vi "CleanHandler.constructor.vi"(0 "name":string, 2 "data in":string, 5 "error in(no error)":errorcluster) -> (14 "i ref out":refnum<vi>, 16 "data out":string, 19 "error out":errorcluster)   [LabVIEW 2014, in "CleanHandler.lvlib"]
doc: "A class handling a couple of DS345 (or a similar AFG) objects for sideband free cleaning by dipole excitation in the precision trap. Most of the DS345 are used to output a sine wave at the desired frequency. The amplitude of these DS345 is modulated by a Gaussian waveform that is generated by the first DS345 in the list of used devices. An instance of the CleanHandler instantiates its function generators when it is created. The function generators to be used are specified in the database.\n\nauthor: Dietrich Beck, GSI\n\nLicense Agreement for this software:\n\nCopyright (C)\nGesellschaft für Schwerionenforschung, GSI\nPlanckstr. 1\n64291 Darmstadt\nGermany\n\nContact: D.Beck@gsi.de \n\nThis program is free software; you can redistribute it and/or modify it under the terms of the \nGNU General Public License as published by the Free Software Foundation; either version 2 of \nthe license, or (at your option) any later version.\n\nThis program is distributed in the hope that it will be useful, but WITHOUT ANY WARRANTY; \nwithout even the implied warranty of MERCHANTABILITY or FITNESS FOR A PARTICULAR PURPOSE. See the GNU General License for more details (http://www.gnu.org).\n\nGesellschaft für Schwerionenforschung, GSI\nPlanckstr. 1, 64291 Darmstadt, Germany\nFor all questions and ideas contact: M.Richter@gsi.de, H.Brand@gsi.de or D.Beck@gsi.de.\nLast update: 16-JUN-2004"
uses:
  CleanHandler.lvlib
  CS_Core/BaseProcess/BaseProcess.lvlib
  CS_Core/CSSystem/CSSystemLib/CSSystemLib.lvlib
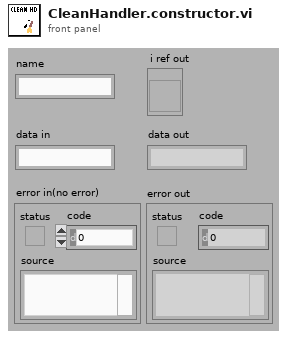
[diagram p1: front panel]
types:
  T1 = enum16{"SetAttribute", "GetAttribute", "CreateAttribute", "DestroyAttribute", "DestroyAllAtributes"}
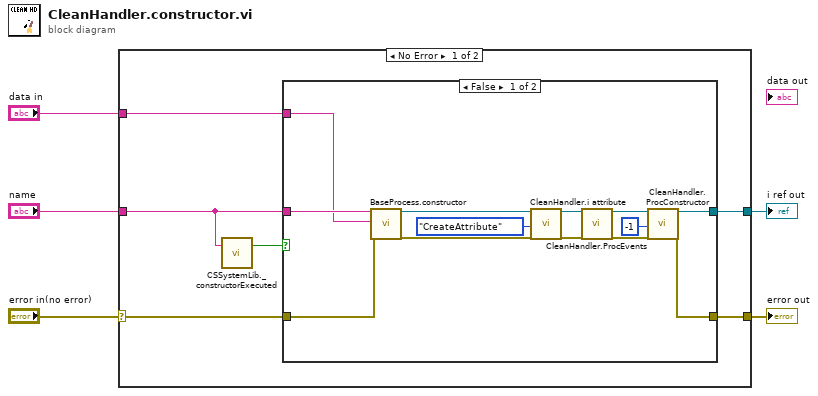
[diagram p0: block diagram]
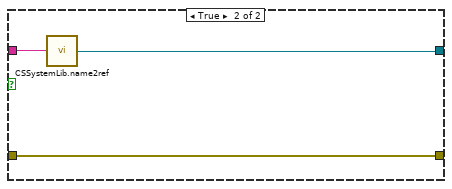
[diagram p2: hidden frame]
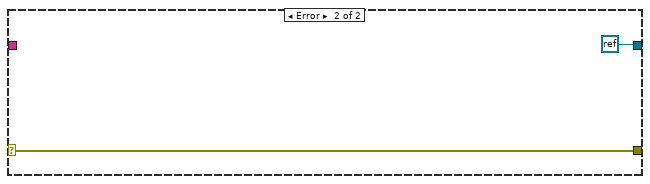
[diagram p3: hidden frame]
diagram:
  n1 = case shown="No Error" "error in(no error)" {
    selector: "error in(no error)" -> [w8 w29]
    tunnel: "name" -> [w6 _]
    tunnel: [w11 refnum<k0> refnum] -> w4
    tunnel: [w10 w29] -> w3
    tunnel: "data in" -> [w9 _]
    frame No Error {
      n2 = call "CSSystemLib._constructorExecuted.vi"("name"=w6) -> ("constructor executed?"=w7:bool)  [unwired: 18 in]
      n3 = case shown="False" w7 {
        tunnel: w8 -> [w24 w27]
        tunnel: w6 -> [w20 w26]
        tunnel: [w14 w25] -> w11
        tunnel: [w13 w27] -> w10
        tunnel: w9 -> [w12 _]
        frame False {
          n4 = call "BaseProcess.constructor.vi"("name"=w20, "data in"=w12, "error in (no error)"=w24) -> ("i ref out"=w23:refnum<vi>, "error out"=w22:errorcluster)  [unwired: 14 in, 1 out]
          n5 = call "CleanHandler.i attribute.vi"("VI Refnum"=w23, "Action"=T1."CreateAttribute", "error in (no error)"=w22) -> ("VI Refnum out"=w19:refnum<vi>, "error out"=w18:errorcluster)  [unwired: 14 in, 1 out]
          n6 = call "CleanHandler.ProcEvents.vi"("i ref in"=w19, "error in"=w18) -> ("i ref out"=w17:refnum<vi>, "error out"=w16:errorcluster)  [unwired: 16 in]
          n7 = call "CleanHandler.ProcConstructor.vi"("i ref in"=w17, "ms timeout (100)"=-1, "error in (no error)"=w16) -> ("i ref out"=w14:refnum<vi>, "error out"=w13:errorcluster)  [unwired: 14 in, 1 out]
        }
        frame True {
          n8 = call "CSSystemLib.name2ref.vi"("name"=w26) -> ("obj refnum"=w25:refnum<vi>)
        }
      }
    }
    frame Error {
    }
  }
  "i ref out" <- w4
  "error out" <- w3
